vi "Microwave Control Panel (No Objects).vi"(8 "error in (no error)":errorcluster) -> (0 "error out":errorcluster)   [LabVIEW 2012]
uses:
  Global/GPIB Type Def.ctl
  Agilent PSG MXG Series/Agilent PSG MXG Series.lvlib
panel:
  in  "Microwave Generator":T1={"Name"="Microwave Gen.", "bus"=0.0, "GPIB"=19.0, "GPIB as string"="19", "byte"=1024, "VISA Resource Name"="GPIB0::19::INSTR"}
  out "Ready when blinking":bool
  out "Amplitude Mode":enum16{"Fixed", "Stepped Sweep", "List Sweep"}(ring)
  out "Frequency Mode":T2(ring)
  in  "Amplitude Mode Set":enum16{"Fixed", "Stepped Sweep", "List Sweep"}(ring)
  in  "Frequency Mode Set":T2(ring)
  in  "Copy actual to set":bool
  in  "Populate fields with member data":bool
  out "Dwell":dbl[unit]
  out "Points":i32
  in  "Dwell Set":dbl[unit]
  in  "Points Set":i32
  out "Freq Stop":dbl[unit]
  out "Freq Start":dbl[unit]
  in  "Freq Stop Set":dbl[unit]
  in  "Freq Start Set":dbl[unit]
  out "Amp Stop":dbl
  out "Amp Start":dbl
  in  "Amp Stop Set":dbl
  in  "Amp Start Set":dbl
  out "Amplitude":dbl
  out "Frequency":dbl[unit]
  in  "Amplitude Set":dbl
  in  "Frequency Set":dbl[unit]
  in  "Rf On/Off":bool caption="rf On/Off"
  in  "Exit":bool
  in  "Set":bool
  in  "Read to Control":bool
  in  "Read":bool
  in  "Reset":bool
  # "Microwave Front Panel"
  # "Output Mode"
  # "CW Operation Settings"
  # "Generic Sweep Settings"
  # "dBm"
  # "dBm"
  # "Frequency Sweep Settings"
  # "Amplitude Sweep Settings"
  # "dBm"
  # "dBm"
  # "dBm"
  # "dBm"
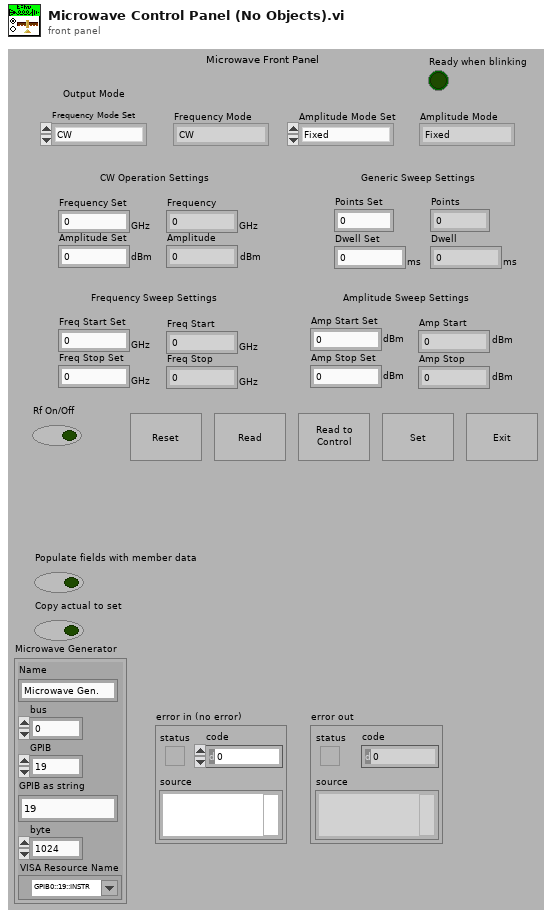
[diagram p1: front panel]
types:
  T1 = typedef "GPIB Type Def.ctl" = cluster{"Name":string, "bus":dbl, "GPIB":dbl, "GPIB as string":string, "byte":i32, "VISA Resource Name":refnum<visa-resource-name>}
  T2 = enum16{"CW", "Fixed", "Stepped Sweep", "List Sweep"}
  T3 = cluster{"Frequency Mode":u16, "Amplitude Mode":u16, "Frequency":dbl[unit], "Amplitude (dBm)":dbl, "Sweep Points":i32, "Sweep Dwell":dbl[unit], "Freq Sweep Start":dbl[unit], "Freq Sweep Stop":dbl[unit], "Amp Sweep Start (dBm)":dbl, "Amp Sweep Stop (dBm)":dbl, "rf on?":bool}
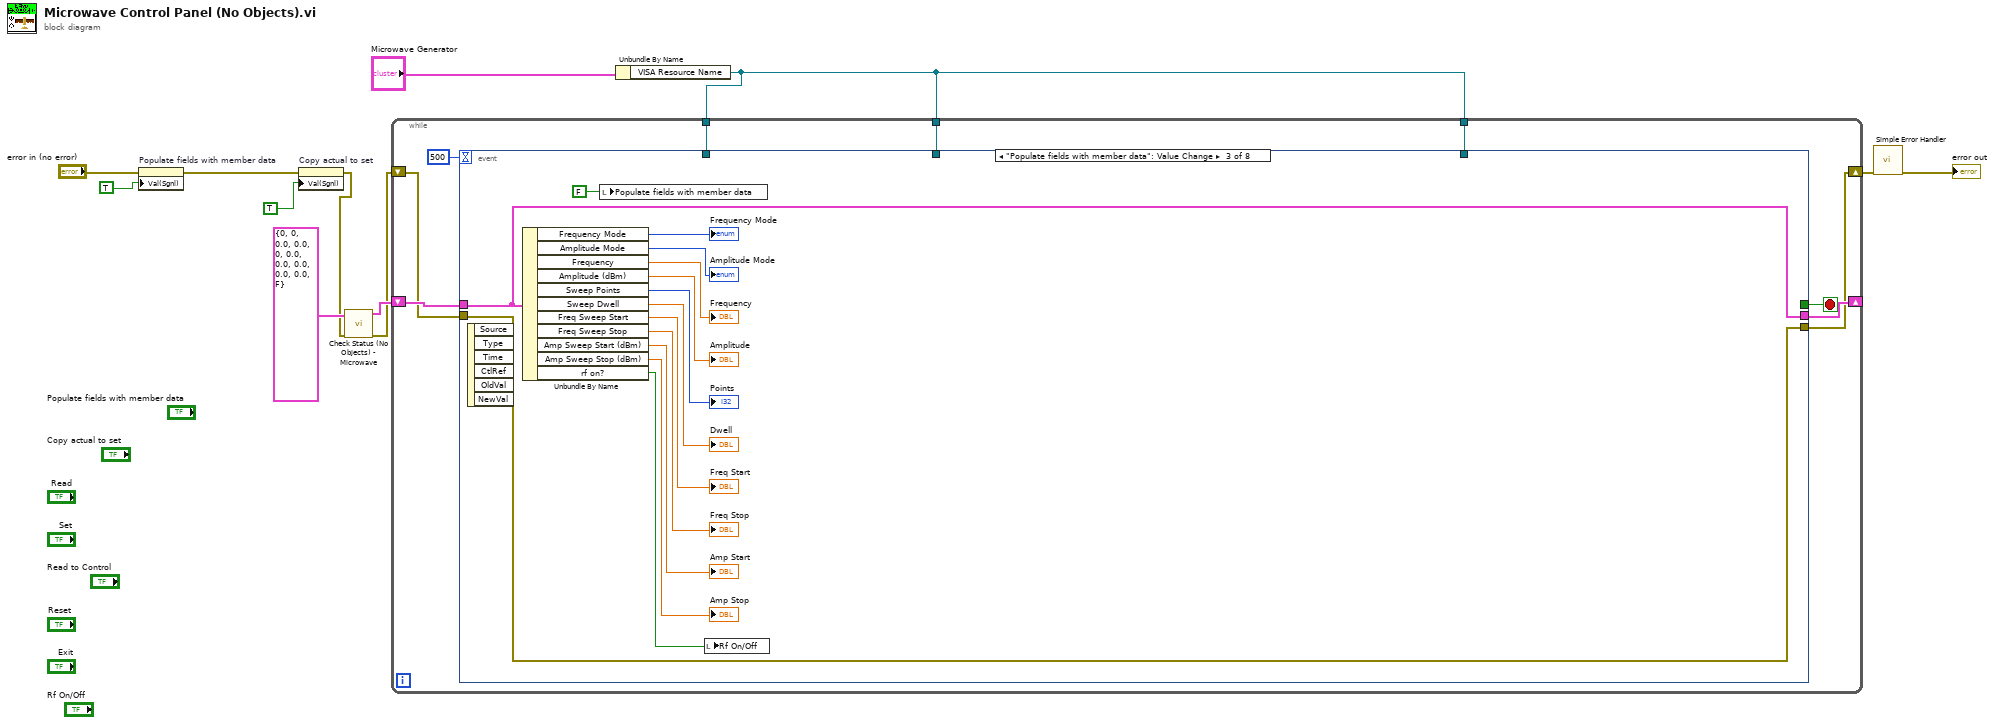
[diagram p0: block diagram]
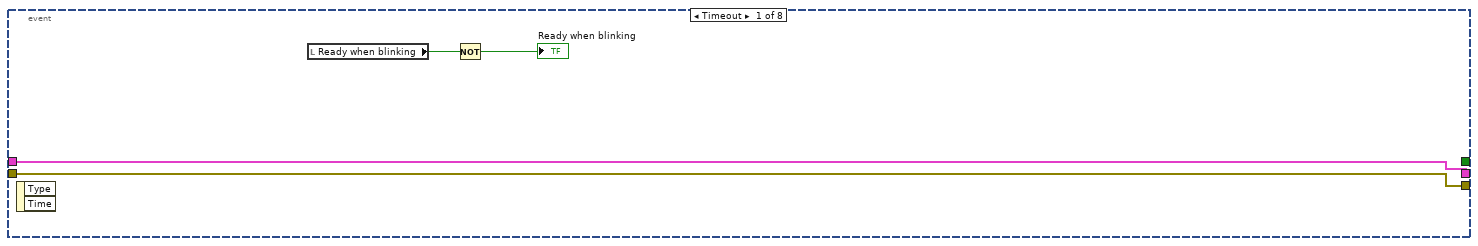
[diagram p2: hidden frame]
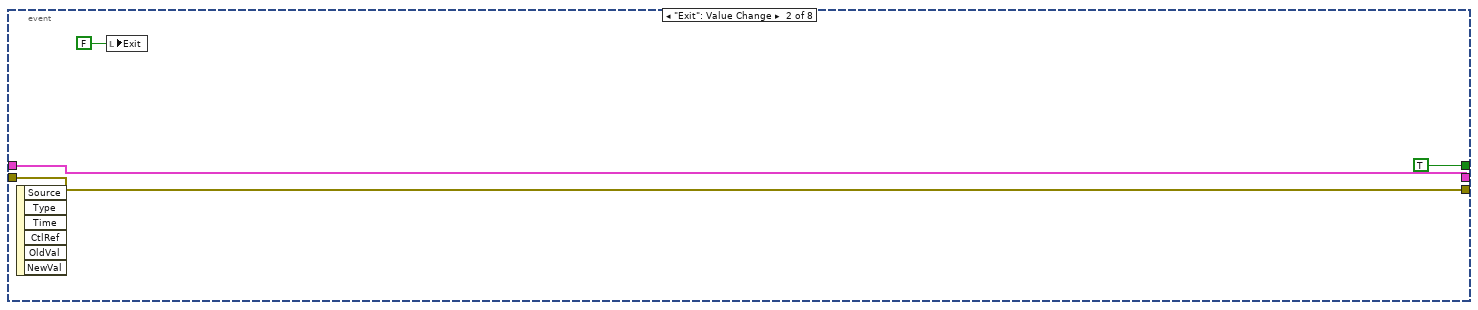
[diagram p3: hidden frame]
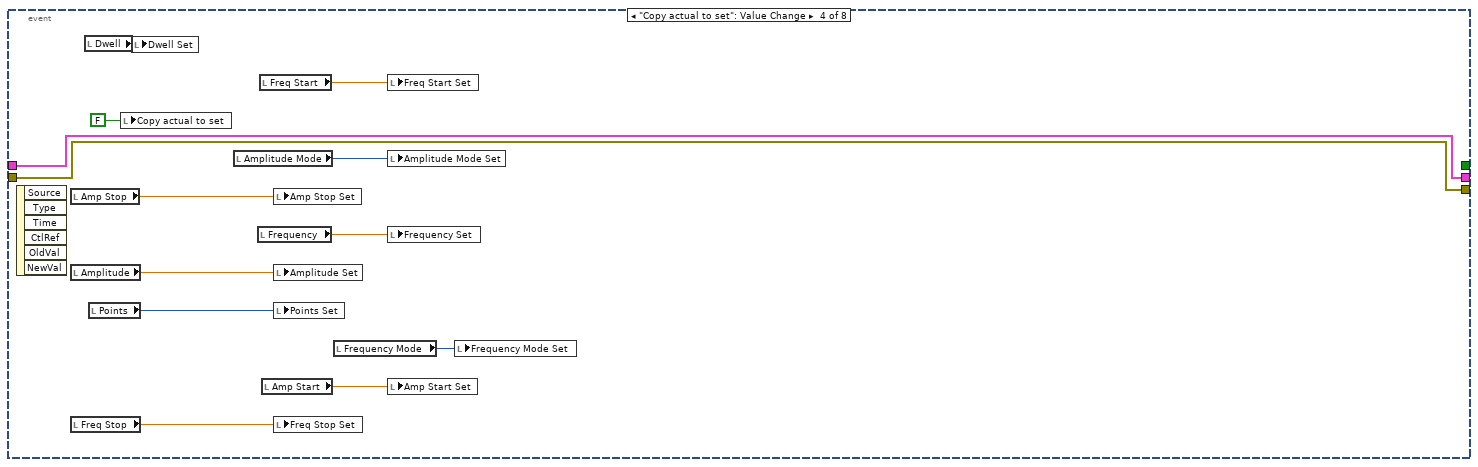
[diagram p4: hidden frame]
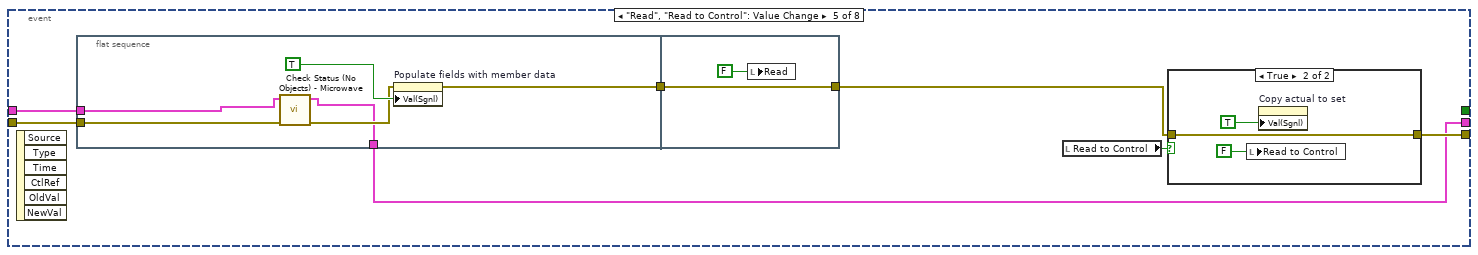
[diagram p5: hidden frame]
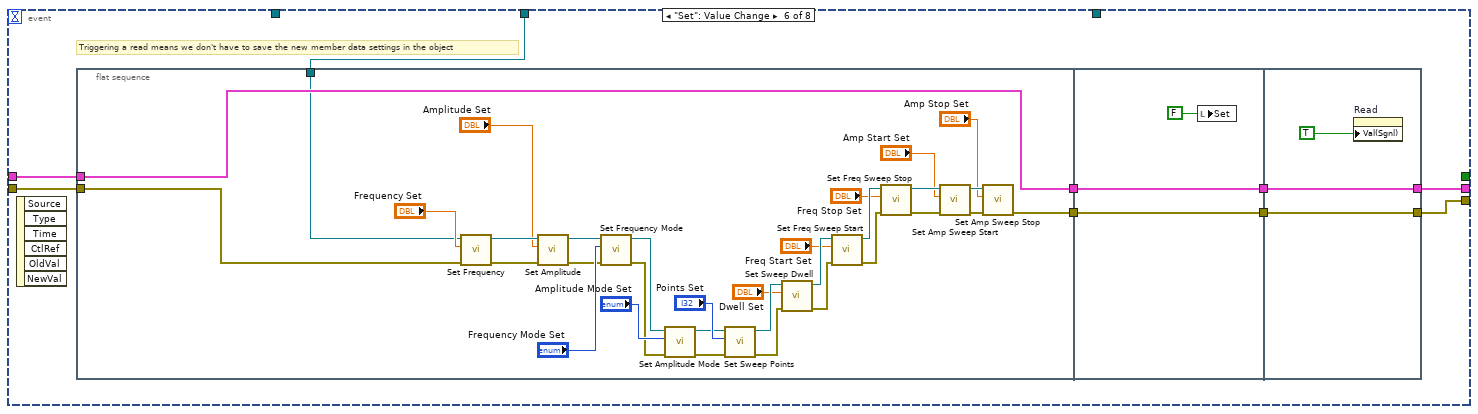
[diagram p7: hidden frame]
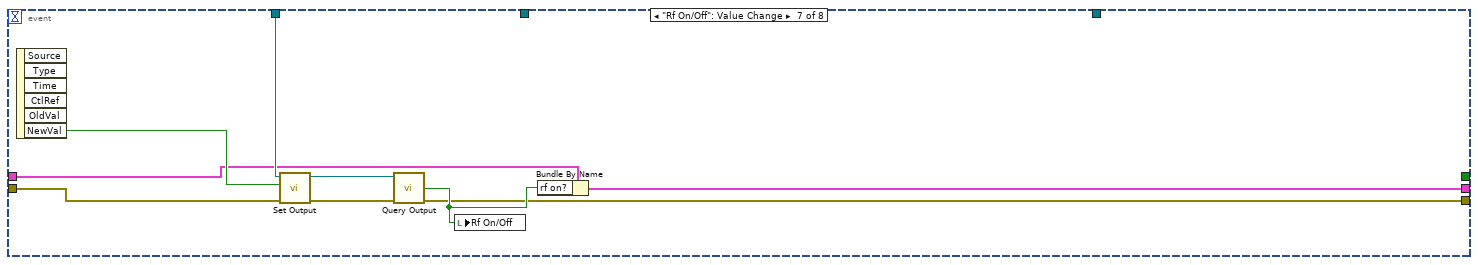
[diagram p8: hidden frame]
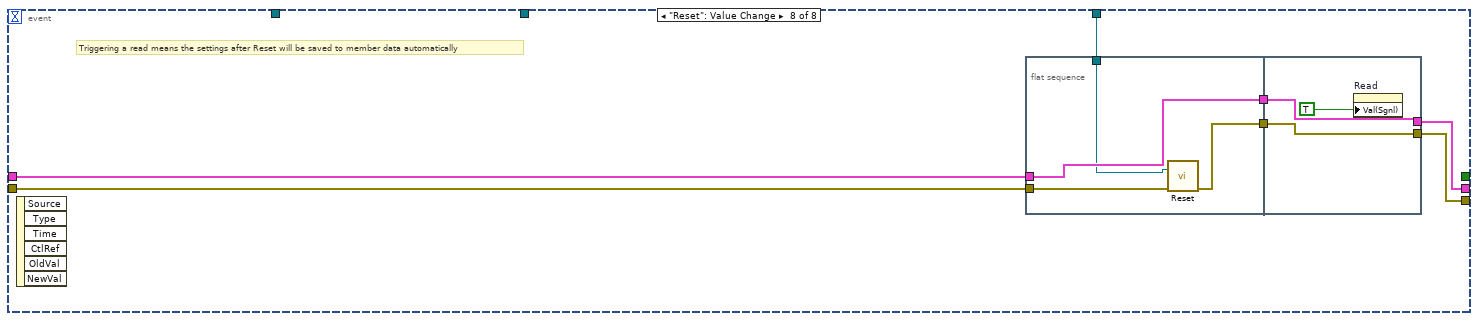
[diagram p9: hidden frame]
diagram:
  n1 = property on="Populate fields with member data" class="Bool (strict)"(error in="error in (no error)", "Val(Sgnl)"=TRUE ("Value (Signaling)")) -> (error out=w10:errorcluster)  [unwired: 1 in, 1 out]
  n2 = property on="Copy actual to set" class="Bool (strict)"(error in=w10, "Val(Sgnl)"=TRUE ("Value (Signaling)")) -> (error out=w3:errorcluster)  [unwired: 1 in, 1 out]
  n3 = call "Check Status (No Objects) - Microwave.vi"("error in (no error)"=w3, "Cluster In"=T3 {"Frequency Mode"=0, "Amplitude Mode"=0, "Frequency"=0.0, "Amplitude (dBm)"=0.0, "Sweep Points"=0, "Sweep Dwell"=0.0, "Freq Sweep Start"=0.0, "Freq Sweep Stop"=0.0, "Amp Sweep Start (dBm)"=0.0, "Amp Sweep Stop (dBm)"=0.0, "rf on?"=FALSE} ("Cluster of class private data")) -> ("error out"=w2:errorcluster, "Cluster Out"=w4:T3)  [unwired: 6 in, 2 out]
  n4 = Unbundle By Name("Microwave Generator") -> ("VISA Resource Name"=w6:refnum<visa-resource-name>)
  n5 = while {
    shift-right: [w19] -> w9
    shift-left: w2 -> [w18]
    shift-right: [w20] -> _
    shift-left: w4 -> [w21]
    tunnel: w6 -> [w15]
    tunnel: w6 -> [w14]
    tunnel: w6 -> [w13]
    stop <- w17 stop-if-true
    n6 = event shown="[2] \"Populate fields with member data\": Value Change" {
      selector: _ -> [_ _ _ _ _ _ _ _]
      dyn-events: _ -> [_ _ _ _ _ _ _ _]
      timeout: 500 -> [_ _ _ _ _ _ _ _]
      tunnel: w21 -> [w25 w29 w32 w56 w58 w84 w123 w138]
      tunnel: [w25 w29 w32 w56 w57 w83 w131 w137] -> w20
      tunnel: [w24 w28 w43 w55 w59 w81 w124 w135] -> w19
      tunnel: w18 -> [w24 w28 w43 w55 w62 w82 w125 w136]
      tunnel: [_ TRUE ("exit") _ _ _ _ _ _] -> w17
      tunnel: w15 -> [_ _ _ _ _ w76 _ _]
      tunnel: w14 -> [_ _ _ _ _ _ _ w132]
      tunnel: w13 -> [_ _ _ _ _ _ w126 _]
      event Timeout {
        n7 = event-data() -> ()  [unwired: 3 out]
        n8 = local read "Ready when blinking"() -> (w22:bool)
        n9 = Not(x=w22) -> (.not. x?=→"Ready when blinking":bool)
      }
      event "Exit": Value Change {
        n10 = event-data() -> ()  [unwired: 7 out]
        n11 = local write "Exit"(FALSE ("Exit")) -> ()
      }
      event "Populate fields with member data": Value Change {
        n12 = event-data() -> ()  [unwired: 7 out]
        n13 = Unbundle By Name(w32) -> ("Frequency Mode"=→"Frequency Mode":u16, "Amplitude Mode"=→"Amplitude Mode":u16, "Frequency"=→"Frequency":dbl[unit], "Amplitude (dBm)"=→"Amplitude":dbl, "Sweep Points"=→"Points":i32, "Sweep Dwell"=→"Dwell":dbl[unit], "Freq Sweep Start"=→"Freq Start":dbl[unit], "Freq Sweep Stop"=→"Freq Stop":dbl[unit], "Amp Sweep Start (dBm)"=→"Amp Start":dbl, "Amp Sweep Stop (dBm)"=→"Amp Stop":dbl, "rf on?"=w30:bool)
        n14 = local write "Populate fields with member data"(FALSE ("Populate fields with member data")) -> ()
        n15 = local write "Rf On/Off"(w30) -> ()
      }
      event "Copy actual to set": Value Change {
        n16 = event-data() -> ()  [unwired: 7 out]
        n17 = local read "Amp Stop"() -> (w45:dbl)
        n18 = local read "Amplitude"() -> (w51:dbl)
        n19 = local read "Freq Stop"() -> (w47:dbl[unit])
        n20 = local read "Dwell"() -> (w49:dbl[unit])
        n21 = local read "Points"() -> (w50:i32)
        n22 = local write "Copy actual to set"(FALSE ("Copy actual to set")) -> ()
        n23 = local write "Dwell Set"(w49) -> ()
        n24 = local read "Amplitude Mode"() -> (w53:enum16{"Fixed", "Stepped Sweep", "List Sweep"})
        n25 = local read "Frequency"() -> (w52:dbl[unit])
        n26 = local read "Freq Start"() -> (w48:dbl[unit])
        n27 = local read "Amp Start"() -> (w46:dbl)
        n28 = local write "Amp Stop Set"(w45) -> ()
        n29 = local write "Amplitude Set"(w51) -> ()
        n30 = local write "Points Set"(w50) -> ()
        n31 = local write "Freq Stop Set"(w47) -> ()
        n32 = local read "Frequency Mode"() -> (w54:T2)
        n33 = local write "Freq Start Set"(w48) -> ()
        n34 = local write "Amplitude Mode Set"(w53) -> ()
        n35 = local write "Frequency Set"(w52) -> ()
        n36 = local write "Amp Start Set"(w46) -> ()
        n37 = local write "Frequency Mode Set"(w54) -> ()
      }
      event "Read", "Read to Control": Value Change {
        n38 = event-data() -> ()  [unwired: 7 out]
        n39 = flat-sequence {
          tunnel: w58 -> [w69]
          tunnel: w62 -> [w73]
          tunnel: [w70] -> w60
          tunnel: [w68] -> w57
          tunnel: [w74] -> w61
          tunnel: w60 -> [w74]
          frame #0 {
            n40 = call "Check Status (No Objects) - Microwave.vi"("error in (no error)"=w73, "Cluster In"=w69) -> ("error out"=w71:errorcluster, "Cluster Out"=w68:T3)  [unwired: 6 in, 2 out]
            n41 = property on="Populate fields with member data" class="Bool (strict)"(error in=w71, "Val(Sgnl)"=TRUE ("Value (Signaling)")) -> (error out=w70:errorcluster)  [unwired: 1 in, 1 out]
          }
          frame #1 {
            n42 = local write "Read"(FALSE ("Read")) -> ()
          }
        }
        n43 = local read "Read to Control"() -> (w63:bool)
        n44 = case shown="True" w63 {
          tunnel: [w64 w67] -> w59
          tunnel: w61 -> [w64 w67]
          frame False {
          }
          frame True {
            n45 = local write "Read to Control"(FALSE ("Read to Control")) -> ()
            n46 = property on="Copy actual to set" class="Bool (strict)"("Val(Sgnl)"=TRUE ("Value (Signaling)")) -> ()  [unwired: 2 in, 2 out]
          }
        }
      }
      event "Set": Value Change {
        # "Triggering a read means we don't have to save the new member data settings in the object"
        n47 = event-data() -> ()  [unwired: 7 out]
        n48 = flat-sequence {
          tunnel: w84 -> [w87]
          tunnel: w82 -> [w86]
          tunnel: [w87] -> w80
          tunnel: [w88] -> w79
          tunnel: w76 -> [w85]
          tunnel: w80 -> [w119]
          tunnel: w79 -> [w118]
          tunnel: [w119] -> w78
          tunnel: [w118] -> w77
          tunnel: [w121] -> w81
          tunnel: [w122] -> w83
          tunnel: w78 -> [w122]
          tunnel: w77 -> [w121]
          frame #0 {
            n49 = call "Set Frequency.vi"("error in (no error)"=w86, "Frequency"="Frequency Set", "VISA resource name"=w85) -> ("error out"=w109:errorcluster, "VISA resource name out"=w115:refnum<visa-resource-name>)  [unwired: 7 out]
            n50 = call "Set Amplitude.vi"("error in (no error)"=w109, "Amplitude (dBm)"="Amplitude Set", "VISA resource name"=w115) -> ("error out"=w91:errorcluster, "VISA resource name out"=w92:refnum<visa-resource-name>)  [unwired: 7 out]
            n51 = call "Set Frequency Mode.vi"("error in (no error)"=w91, "Frequency Mode"="Frequency Mode Set", "VISA resource name"=w92) -> ("error out"=w93:errorcluster, "VISA resource name out"=w116:refnum<visa-resource-name>)  [unwired: 7 out]
            n52 = call "Set Amplitude Mode.vi"("error in (no error)"=w93, "Amplitude Mode"="Amplitude Mode Set", "VISA resource name"=w116) -> ("error out"=w90:errorcluster, "VISA resource name out"=w89:refnum<visa-resource-name>)  [unwired: 7 out]
            n53 = call "Set Sweep Points.vi"("error in (no error)"=w90, "Number of Sweep Points"="Points Set", "VISA resource name"=w89) -> ("error out"=w108:errorcluster, "VISA resource name out"=w114:refnum<visa-resource-name>)  [unwired: 7 out]
            n54 = call "Set Sweep Dwell.vi"("error in (no error)"=w108, "Sweep Dwell Time"="Dwell Set", "VISA resource name"=w114) -> ("error out"=w107:errorcluster, "VISA resource name out"=w113:refnum<visa-resource-name>)  [unwired: 7 out]
            n55 = call "Set Freq Sweep Start.vi"("error in (no error)"=w107, "Frequency Sweep Start"="Freq Start Set", "VISA resource name"=w113) -> ("error out"=w106:errorcluster, "VISA resource name out"=w112:refnum<visa-resource-name>)  [unwired: 7 out]
            n56 = call "Set Freq Sweep Stop.vi"("error in (no error)"=w106, "Frequency Sweep Stop"="Freq Stop Set", "VISA resource name"=w112) -> ("error out"=w105:errorcluster, "VISA resource name out"=w111:refnum<visa-resource-name>)  [unwired: 7 out]
            n57 = call "Set Amp Sweep Start.vi"("error in (no error)"=w105, "Amplitude Sweep Start (dBm)"="Amp Start Set", "VISA resource name"=w111) -> ("error out"=w104:errorcluster, "VISA resource name out"=w110:refnum<visa-resource-name>)  [unwired: 7 out]
            n58 = call "Set Amp Sweep Stop.vi"("error in (no error)"=w104, "Amplitude Sweep Stop (dBm)"="Amp Stop Set", "VISA resource name"=w110) -> ("error out"=w88:errorcluster)  [unwired: 8 out]
          }
          frame #1 {
            n59 = local write "Set"(FALSE ("Set")) -> ()
          }
          frame #2 {
            n60 = property on="Read" class="Bool (strict)"("Val(Sgnl)"=TRUE ("Value (Signaling)")) -> ()  [unwired: 2 in, 2 out]
          }
        }
      }
      event "Rf On/Off": Value Change {
        n61 = event-data() -> ("NewVal"=w130:bool)  [unwired: 6 out]
        n62 = call "Set Output.vi"("error in (no error)"=w125, "Output On"=w130, "VISA resource name"=w126) -> ("error out"=w128:errorcluster, "VISA resource name out"=w129:refnum<visa-resource-name>)  [unwired: 7 out]
        n63 = call "Query Output.vi"("error in (no error)"=w128, "VISA resource name"=w129) -> ("error out"=w124:errorcluster, "Output On?"=w127:bool)  [unwired: 8 out]
        n64 = local write "Rf On/Off"(w127) -> ()
        n65 = Bundle By Name(cluster=w123, "rf on?"=w127) -> (w131:T3)
      }
      event "Reset": Value Change {
        # "Triggering a read means the settings after Reset will be saved to member data automatically"
        n66 = event-data() -> ()  [unwired: 7 out]
        n67 = flat-sequence {
          tunnel: w138 -> [w142]
          tunnel: w136 -> [w140]
          tunnel: [w142] -> w134
          tunnel: [w141] -> w133
          tunnel: w132 -> [w139]
          tunnel: [w144] -> w135
          tunnel: [w145] -> w137
          tunnel: w134 -> [w145]
          tunnel: w133 -> [w144]
          frame #0 {
            n68 = call "Reset.vi"("error in (no error)"=w140, "VISA resource name"=w139) -> ("error out"=w141:errorcluster)  [unwired: 9 out]
          }
          frame #1 {
            n69 = property on="Read" class="Bool (strict)"("Val(Sgnl)"=TRUE ("Value (Signaling)")) -> ()  [unwired: 2 in, 2 out]
          }
        }
      }
    }
  }
  n70 = call <vilib>:"Simple Error Handler.vi"("error in (no error)"=w9) -> ("error out"=→"error out":errorcluster)  [unwired: 1 in, 7 out]
